vi "Untitled sensor.vi"() -> ()   [LabVIEW 2019]
uses:
  <vilib>/myRIO/Instrument Drivers/Onboard IO/I2C/typedefs/I2C User Configuration.ctl
  <vilib>/myRIO/Instrument Drivers/Onboard IO/I2C/typedefs/I2C Transfer Rate.ctl
  <vilib>/myRIO/Instrument Drivers/Onboard IO/DIO/typedefs/DIO Reference.ctl
  <vilib>/myRIO/Common/Instrument Driver Framework/Utilities/typedefs/myRIO Generic Hardware Reference.ctl
  <vilib>/myRIO/Common/Instrument Driver Framework/Utilities/typedefs/Hardware Version Enum.ctl
  <vilib>/myRIO/Common/Instrument Driver Framework/Utilities/typedefs/myRIO v1.0 Reference.ctl
  <vilib>/myRIO/Common/Instrument Driver Framework/Utilities/typedefs/Generic FPGA Reference.ctl
  <vilib>/myRIO/Common/Instrument Driver Framework/myRIO v1.0/DIO/typedefs/DIO Channels List.ctl
  <vilib>/myRIO/Common/Instrument Driver Framework/myRIO v1.0/DIO/typedefs/DIO Channels Enum.ctl
  <vilib>/userdefined/High Color/nirio_resource_hc.ctl
  <vilib>/Platform/TimedLoop/XDataNode/timing_clust.ctl
  <vilib>/Platform/TimedLoop/XDataNode/nitl_modes.ctl
  <vilib>/Platform/TimedLoop/XDataNode/wakeup.ctl
  <vilib>/myRIO/Common/Instrument Driver Framework/Utilities/vis/Is FPGA Ref Available.vi
  <vilib>/myRIO/Common/Instrument Driver Framework/myRIO v1.0/DIO/vis/myRIO v1.1 Open DIO.vi
  <vilib>/myRIO/Common/Instrument Driver Framework/Utilities/vis/Validate Channels.vi
  <vilib>/myRIO/Common/Instrument Driver Framework/myRIO v1.0/DIO/vis/myRIO v1.0 Reserve DIO.vi
  <vilib>/myRIO/Common/Instrument Driver Framework/myRIO v1.0/Resource Manager/vis/myRIO v1.0 Reserve Channel List.vi
  <vilib>/myRIO/Common/Instrument Driver Framework/myRIO v1.0/DIO/vis/myRIO v1.0 Build MUX Configuration DIO.vi
  <vilib>/myRIO/Common/Instrument Driver Framework/myRIO v1.0/Resource Manager/vis/myRIO v1.0 Reserve Channel.vi
  <vilib>/myRIO/Common/Instrument Driver Framework/myRIO v1.0/Resource Manager/vis/myRIO v1.0 Unreserve Channel.vi
  <vilib>/myRIO/Common/Instrument Driver Framework/myRIO v1.0/Resource Manager/vis/myRIO v1.0 Create Configuration List.vi
  <vilib>/myRIO/Common/Instrument Driver Framework/myRIO v1.0/Resource Manager/vis/myRIO v1.0 Build Mutex Name.vi
  <vilib>/Utility/VariantDataType/GetNumericInfo.vi
  <vilib>/Utility/error.llb/Error Cluster From Error Code.vi
  <vilib>/myRIO/Common/Instrument Driver Framework/myRIO v1.0/myRIO v1.1 Open.vi
  <vilib>/myRIO/Common/Instrument Driver Framework/Utilities/vis/IO Manager.vi
  <vilib>/myRIO/Common/Instrument Driver Framework/Utilities/vis/Configuration Manager.vi
  <vilib>/myRIO/Common/Instrument Driver Framework/myRIO v1.0/Resource Manager/vis/myRIO v1.0 Configure IO.vi
  <vilib>/myRIO/Common/Instrument Driver Framework/myRIO v1.0/myRIO v1.0 Close.vi
  <vilib>/myRIO/Common/Instrument Driver Framework/myRIO v1.0/DIO/vis/myRIO v1.0 Write DIO.vi
  <vilib>/myRIO/Common/Instrument Driver Framework/myRIO v1.0/I2C/vis/myRIO v1.0 Configure I2C.vi
  <vilib>/myRIO/Common/Instrument Driver Framework/myRIO v1.0/I2C/vis/myRIO v1.0 Write I2C.vi
  <vilib>/myRIO/Common/Instrument Driver Framework/myRIO v1.0/I2C/vis/myRIO v1.0 Read I2C.vi
  Global.vi
  <vilib>/myRIO/Express VI/Onboard IO/DO/DO Express VI.xnode
  <vilib>/myRIO/Instrument Drivers/Onboard IO/DIO/vis/myRIO DIO Open.xnode
  <vilib>/platform/TimedLoop/XDataNode/XDataNode.xnode
  <vilib>/myRIO/Instrument Drivers/Onboard IO/I2C/I2C.lvlib
  <vilib>/myRIO/Instrument Drivers/Onboard IO/DIO/DIO.lvlib
  <vilib>/Platform/TimedLoop/XDataNode/XDNodeRunTimeDep.lvlib
  <vilib>/Analysis/NI_AAL_SigProc.lvlib
  <vilib>/ptbypt/NI_PtbyPt.lvlib
panel:
  out "Signal with envelopes":dbl[](graph)
  in  "Tab Control 2":enum32{"Graph", "Filter controls"}(tab)
  out "error out":errorcluster
  out "Sensors data":T1(graph)
  in  "Sensor Tare":bool
  in  "Tare sensor":dbl
  in  "error in (no error)":errorcluster
  in  "Width":i32(slide)=10 scale=0.0..500.0
  in  "Threshold":dbl(slide)=4.897959183673464 scale=-60.0..60.0
  out "Locations":dbl[](array[numeric])
  out "element":dbl
  out "size(s)":i32
  in  "Ts":dbl=1e-05
  in  "Tf":dbl=0.01 format="%#_13g"
  in  "Tf 2":dbl=0.01
  in  "Ts 2":dbl=1e-05
  in  "sample length":i32=100
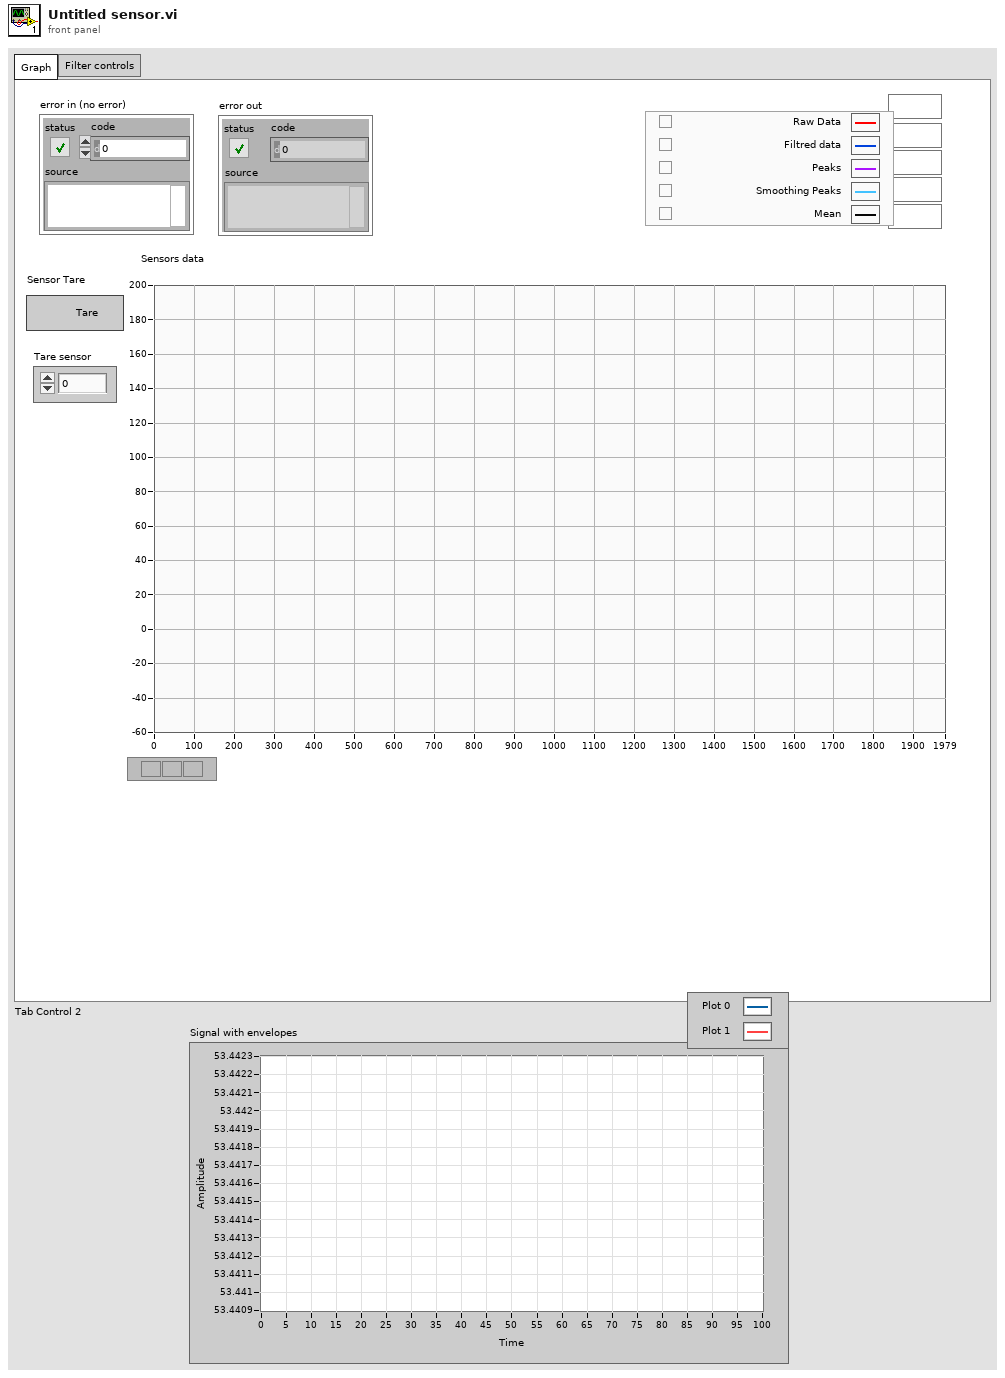
[diagram p1: front panel]
types:
  T1 = cluster{dbl, "yf1":dbl, dbl, "mean":dbl, "mean":dbl}
  T2 = cluster{"yf1":dbl, "yf1":dbl, dbl, "mean":dbl, dbl}[]
  T3 = typedef "DIO.lvlib/DIO Reference.ctl" = cluster{"myRIO Reference":T4, "DIO Channels List":T8}
  T4 = typedef "myRIO Generic Hardware Reference.ctl" = cluster{"myRIO Model":T5, "myRIO Hardware Reference":T6}
  T5 = typedef "Hardware Version Enum.ctl" = enum16{"Unknown", "myRIO-1900", "myRIO-1950", "roboRIO", "NI ELVIS RIO CM", "ELVIS III"}
  T6 = typedef "myRIO v1.0 Reference.ctl" = cluster{"Generic FPGA Reference":T7, "Allow multiple opens":bool}
  T7 = typedef "Generic FPGA Reference.ctl" = refnum<k20>
  T8 = typedef "DIO Channels List.ctl" = T9[]
  T9 = typedef "DIO Channels Enum.ctl" = enum16{"Not Connected", "C/DIO0", "C/DIO1", "C/DIO2", "C/DIO3", "C/DIO4", "C/DIO5", "C/DIO6", "C/DIO7", "A/DIO0", "A/DIO1", "A/DIO2", "A/DIO3", "A/DIO4", "A/DIO5", "A/DIO6", "A/DIO7", "A/DIO8", "A/DIO9", "A/DIO10", "A/DIO11", "A/DIO12", "A/DIO13", "A/DIO14", "A/DIO15", "A/DIO16", "A/DIO17", "A/DIO18", "A/DIO19", "B/DIO0", "B/DIO1", "B/DIO2", "B/DIO3", "B/DIO4", "B/DIO5", "B/DIO6", "B/DIO7", "B/DIO8", "B/DIO9", "B/DIO10", "B/DIO11", "B/DIO12", "B/DIO13", "B/DIO14", "B/DIO15", "B/DIO16", "B/DIO17", "B/DIO18", "B/DIO19", "LED0", "LED1", "LED2", "LED3", "Button0", "DIO/DIO0", "DIO/DIO1", "DIO/DIO2", "DIO/DIO3", "DIO/DIO4", "DIO/DIO5", "DIO/DIO6", "DIO/DIO7", "DIO/DIO8", "DIO/DIO9", "SPI/CS0", "SPI/CS1", "SPI/CS2", "SPI/CS3", "LED RADIO (Green)", "LED RADIO (Red)", "LED COMM (Green)", "LED COMM (Red)", "LED MODE (Green)", "LED MODE (Red)"}
  T10 = typedef "nirio_resource_hc.ctl" = tag
  T11 = typedef "XDNodeRunTimeDep.lvlib/timing_clust.ctl" = cluster{"Expected End [f-1]":u64, "Actual End [f-1]":u64, "Finished Late? [f-1]":bool, "Expected End [i-1]":u64, "Actual End [i-1]":u64, "Finished Late? [i-1]":bool, "Expected Start [i]":u64, "Actual Start [i]":u64, "Expected Start [f]":u64, "Actual Start [f]":u64, "Source Name":string, "Structure Name":string, "Period":i64, "Deadline":i64, "Offset":i64, "Start":i64, "Priority":i32, "Timeout":i32, "Mode":T12, "Wakeup Reason":T13, "Error":errorcluster, "Source Type":string, "Secondary Source Type":string, "Global End Time":u64, "Global Start Time":u64, "Frame Duration":u64, "Iteration Duration":u64, "Assigned CPU":i32, "I/O Scan Engine Mode":u32}
  T12 = typedef "XDNodeRunTimeDep.lvlib/nitl_modes.ctl" = enum32{"No Change", "Process missed periods, maintain original phase", "Discard missed periods, maintain original phase", "Process missed periods, ignore original phase", "Discard missed periods, ignore original phase"}
  T13 = typedef "XDNodeRunTimeDep.lvlib/wakeup.ctl" = enum32{"Normal", "Aborted", "Asynchronous wakeup", "Timing source error", "Timed loop error", "Timeout"}
  T14 = typedef "I2C.lvlib/I2C User Configuration.ctl" = cluster{"I2C Transfer Rate":T15}
  T15 = typedef "I2C.lvlib/I2C Transfer Rate.ctl" = enum16{"Standard mode (100 kbps)", "Fast mode (400 kbps)"}
  T16 = typedef "I2C.lvlib/I2C Reference.ctl" = cluster{"myRIO Reference":T4, "I2C Channels Enum":T17, "I2C Configuration":T18}
  T17 = typedef "I2C Channels Enum.ctl" = enum16{"Not Connected", "A/I2C", "B/I2C", "I2C/I2C"}
  T18 = typedef "I2C.lvlib/I2C Configuration.ctl" = cluster{"I2C Transfer Rate":T15}
  T19 = cluster{dbl, "yf1":dbl, dbl, "yf":dbl, "mean":dbl}
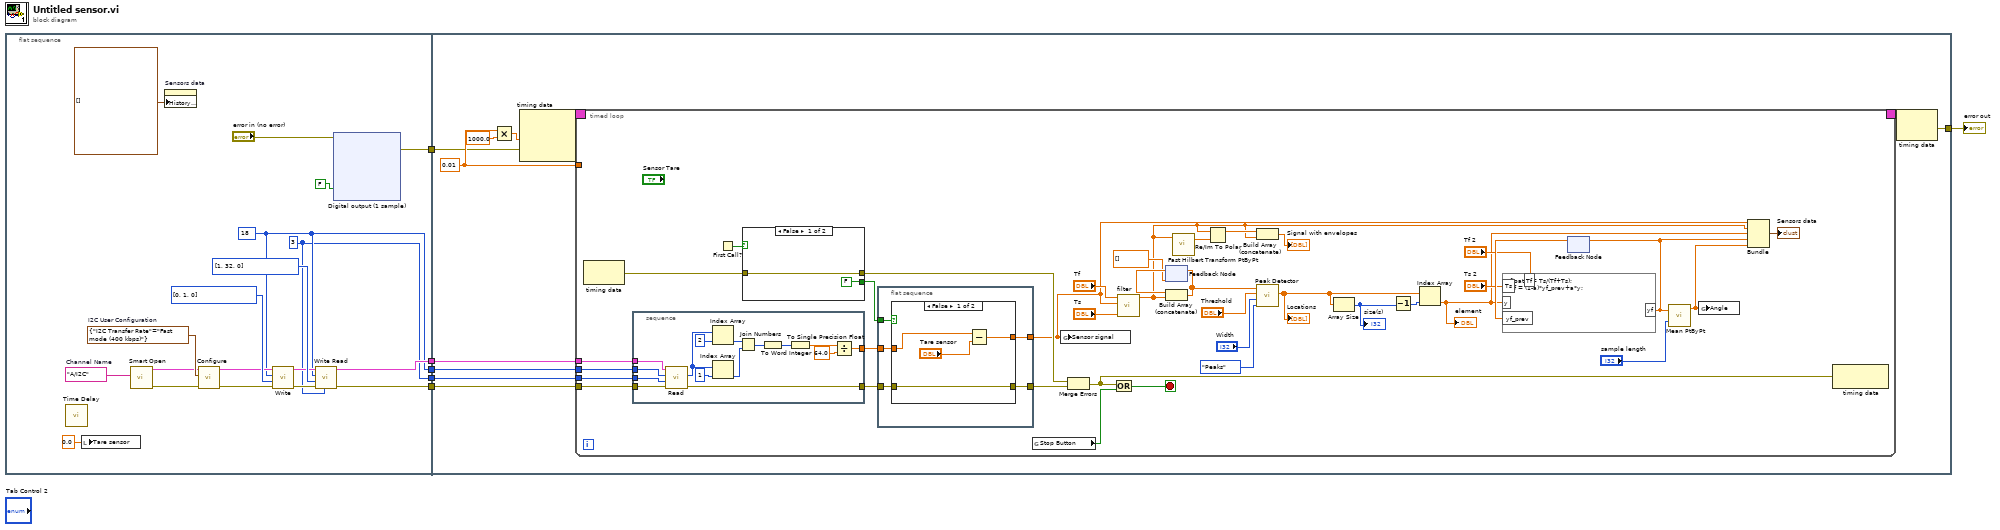
[diagram p0: block diagram]
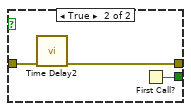
[diagram p2: hidden frame]
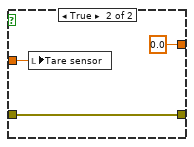
[diagram p3: hidden frame]
diagram:
  n1 = flat-sequence {
    tunnel: [w21] -> w5
    tunnel: [w10] -> w4
    tunnel: [w9] -> w3
    tunnel: [w8] -> w2
    tunnel: [w7] -> w1
    tunnel: [w66] -> w6
    tunnel: w5 -> [w65]
    tunnel: w4 -> [w64]
    tunnel: w3 -> [w63]
    tunnel: w2 -> [w62]
    tunnel: w1 -> [w61]
    frame #0 {
      w8 = u8 18 ("Slave Address (7-bit)")
      w18 = T14 {"I2C Transfer Rate"=enum."Fast mode (400 kbps)"}  # I2C User Configuration
      w13 = tag "A/I2C"  # Channel Name
      w7 = u32 3 ("Byte Count")
      n2 = call "Time Delay"() -> ()  [unwired: 11 in, 1 out]
      n3 = local write "Tare sensor"(0.0 ("Tare sensor 1")) -> ()
      n4 = call <vilib>:"Smart Open.vi"("Channel Name"=w13) -> ("error out"=w11:errorcluster, "I2C Ref Out"=w12:T16)  [unwired: 9 in]
      n5 = property on="Sensors data" class="WFChart (strict)"("History Data"=T2 []) -> ()  [unwired: 2 in, 2 out]
      n6 = call <vilib>:"Configure.vi"("error in (no error)"=w11, "I2C User Configuration"=w18, "I2C Ref In"=w12) -> ("error out"=w15:errorcluster, "I2C Ref Out"=w14:T16)  [unwired: 7 in]
      n7 = call <vilib>:"Write.vi"("error in (no error)"=w15, "Bytes to Write"=u8[] [0, 1, 0], "Slave Address (7-bit)"=w8, "I2C Ref In"=w14) -> ("error out"=w17:errorcluster, "I2C Ref Out"=w16:T16)  [unwired: 6 in]
      n8 = call <vilib>:"Write Read.vi"("Byte Count"=w7, "error in (no error)"=w17, "Bytes to Write"=u8[] [1, 32, 0], "Slave Address (7-bit)"=w8, "I2C Ref In"=w16) -> ("error out"=w9:errorcluster, "I2C Ref Out"=w10:T16)  [unwired: 3 in, 1 out]
      n9 = xnode "Digital output (1 sample)"("A/DIO10 (Pin 31)"=FALSE, "error in (no error)"="error in (no error)") -> ("error out"=w21:errorcluster)
    }
    frame #1 {
      w67 = 0.01
      n10 = Multiply(x=w67, y=1000.0) -> (x*y=w68:dbl)
      n11 = node-c288(w68, w65) -> (w71:T11)  [unwired: 1 in]
      n12 = timed-loop {
        timing: w71 -> [_]
        timing-out: [_] -> w70
        tunnel: w67 -> [_]
        tunnel: w64 -> [w75]
        tunnel: w63 -> [w74]
        tunnel: w62 -> [w73]
        tunnel: w61 -> [w72]
        stop <- w91 stop-if-true
        n13 = node-c288() -> (w83:errorcluster)  [unwired: 1 in]
        n14 = stacked-sequence {
          tunnel: [w138] -> w109
          tunnel: [w134] -> w85
          tunnel: w75 -> [w137]
          tunnel: w74 -> [w136]
          tunnel: w73 -> [w133]
          tunnel: w72 -> [w132]
          frame #0 {
            n15 = call <vilib>:"Read.vi"("error in (no error)"=w136, "Byte Count"=w132, "Slave Address (7-bit)"=w133, "I2C Ref In"=w137) -> ("error out"=w134:errorcluster, "Bytes Read"=w135:u8[])  [unwired: 4 in, 1 out]
            n16 = Index Array(array=w135, index=2) -> (element=w139:u8)
            n17 = Index Array(array=w135, index=1) -> (element=w140:u8)
            n18 = Join Numbers(hi=w139, lo=w140) -> ((hi.lo)=w141:u16)
            n19 = To Word Integer(number=w141) -> (16bit integer=w142:i16)
            n20 = To Single Precision Float(number=w142) -> (single precision float=w143:sgl)
            n21 = Divide(x=w143, y=sgl 64.0) -> (x/y=w138:sgl)
          }
        }
        n22 = First Call?() -> (First Call?: T/F=w93:bool)
        n23 = case shown="False" w93 {
          tunnel: [FALSE ("initialize: T/F") w114] -> w92
          tunnel: w83 -> [w110 w113]
          tunnel: [w110 w112] -> w88
          frame False {
          }
          frame True {
            n24 = call "Time Delay2"("error in (no error)"=w113) -> ("error out"=w112:errorcluster)  [unwired: 10 in]
            n25 = First Call?() -> (First Call?: T/F=w114:bool)
          }
        }
        n26 = flat-sequence {
          tunnel: [w124] -> w86
          tunnel: w109 -> [w123]
          tunnel: w92 -> [w122]
          tunnel: w85 -> [w121]
          tunnel: [w120] -> w84
          frame #0 {
            n27 = case shown="False" w122 {
              tunnel: [w128 0.0] -> w124
              tunnel: w123 -> [w127 w130]
              tunnel: w121 -> [w125 w129]
              tunnel: [w125 w129] -> w120
              frame False {
                n28 = Subtract(x=w127, y="Tare sensor") -> (x-y=w128:dbl)
              }
              frame True {
                n29 = local write "Tare sensor"(w130) -> ()
              }
            }
          }
        }
        n30 = global read "Global.vi" "Stop Button"() -> (w90:bool)
        n31 = global write "Global.vi" "Sensor signal"(w86) -> ()
        n32 = Merge Errors(w88, w84) -> (w87:errorcluster)
        n33 = Or(x=w87, y=w90) -> (x .or. y?=w91:bool)
        n34 = call "filter.vi"("Ts"="Ts", "y1"=w86, "Tf"="Tf") -> ("yf1"=w77:dbl)  [unwired: 7 in, 1 out]
        n35 = feedback #1(dbl[] []) -> (w106:dbl[])
        n36 = Build Array (concatenate)(w106, w77) -> (w101:dbl[])
        n37 = feedback-in #1(w101) -> ()
        n38 = call <vilib>:"Fast Hilbert Transform PtByPt.vi"("x"=w77) -> ("Hilbert{X}"=w79:dbl[])  [unwired: 3 in, 1 out]
        n39 = Re/Im To Polar(2:w79, 3:w77) -> (1:w78:dbl[])  [unwired: 1 out]
        n40 = Build Array (concatenate)(w78, w77) -> (→"Signal with envelopes":dbl[])
        n41 = call <vilib>:"Peak Detector.vi"("peaks/valleys"=enum32{"Peaks", "Valleys"}."Peaks", "width"="Width", "threshold"="Threshold", "X"=w101) -> ("Amplitudes"=w94:dbl[])  [unwired: 3 in, 4 out]
        "Locations" <- w94
        n42 = Array Size(array=w94) -> (size(s)=w99:i32)
        "size(s)" <- w99
        n43 = Decrement(x=w99) -> (x-1=w100:i32)
        n44 = Index Array(array=w94, index=w100) -> (element=w82:dbl)
        "element" <- w82
        n45 = feedback #2() -> (w98:dbl)  [unwired: 1 in]
        n46 = formula code="float a = Ts/(Tf+Ts);\nyf = (1-a)*yf_prev+a*y;"("Tf"="Tf 2", "Ts"="Ts 2", "y"=w82, "yf_prev"=w98) -> ("yf"=w80:dbl)
        n47 = feedback-in #2(w80) -> ()
        n48 = call <vilib>:"Mean PtByPt.vi"("x"=w80, "sample length"="sample length") -> ("mean"=w81:dbl)  [unwired: 2 in, 1 out]
        n49 = global write "Global.vi" "Angle"(w81) -> ()
        n50 = Bundle(w86, "yf1"=w77, w82, "yf"=w80, "mean"=w81) -> (→"Sensors data":T19)  [unwired: 1 in]
        n51 = node-c288(w87) -> ()  [unwired: 1 out]
      }
      n52 = node-c288(w70) -> (w66:errorcluster)
    }
  }
  "error out" <- w6
